vi "JSON Path Const.vi"(1 "JSON Path":T1) -> (0 "resulting array":string[](array[string]))   [LabVIEW 2017, in "MachineLearning.lvlib"]
uses:
  MachineLearning.lvlib
  TypeDefs/JSONpath.ctl
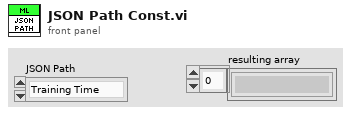
[diagram p1: front panel]
types:
  T1 = typedef "MachineLearning.lvlib/JSONpath.ctl" = enum16{"Training Time", "All Models", "Feature Manipulation", "Anomaly Detection", "Clustering", "Classification", "Custom Info"}
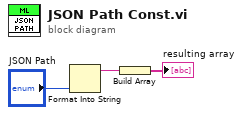
[diagram p0: block diagram]
diagram:
  n1 = Format Into String("JSON Path") -> (resulting string=w3:string)  [unwired: 3 in, 1 out]
  n2 = Build Array(w3) -> (→"resulting array":string[])
